vi "test-path-planner-sample.vi"() -> ()   [LabVIEW 2019]
uses:
  <vilib>/Rock Robotics/WPI/ThirdParty/MJansen/PathPlanner/PathPlannerTrajectory.ctl
  <vilib>/Rock Robotics/WPI/ThirdParty/MJansen/PathPlanner/PathPlannerState.ctl
  <vilib>/Rock Robotics/WPI/ThirdParty/JAS_Junk/TrajLib/TypeDef/ROTATION2D.ctl
  <vilib>/Rock Robotics/WPI/ThirdParty/JAS_Junk/TrajLib/TypeDef/TRAJ_STATE.ctl
  <vilib>/Rock Robotics/WPI/ThirdParty/JAS_Junk/TrajLib/TypeDef/POSE2D.ctl
  <vilib>/Rock Robotics/WPI/ThirdParty/JAS_Junk/TrajLib/TypeDef/TRANSLATION2D.ctl
  <vilib>/Rock Robotics/WPI/ThirdParty/MJansen/PathPlanner/PathPlannerWaypoint.ctl
  <vilib>/Rock Robotics/WPI/ThirdParty/JAS_Junk/TrajLib/Util_ApproxEquals.vi
  <vilib>/Rock Robotics/WPI/ThirdParty/MJansen/PathPlanner/PathPlanner.lvlib
  <vilib>/Rock Robotics/WPI/ThirdParty/JAS_Junk/TrajLib/Trajectory_Library.lvlib
  <vilib>/Analysis/NI_AALBase.lvlib
panel:
  in  "Tab Control":T1(tab)
  in  "Max Velocity":dbl=3.0
  in  "Max Acceleration":dbl=2.0
  in  "stop":bool
  in  "Reversed":bool
  out "PathPlannerWayPoints":T2[](array[typedef]) {"HolonomicRotation"."SIN" format="%13.4f"; "HolonomicRotation"."COS" format="%13.4f"; "HolonomicRotation"."VALUE" format="%13.4f"; "NextControl"."Y" format="%14.3f"; "NextControl"."X" format="%14.3f"; "PrevControl"."Y" format="%14.3f"; "PrevControl"."X" format="%14.3f"; "AnchorPoint"."Y" format="%14.3f"; "AnchorPoint"."X" format="%14.3f"}
  in  "Path FileName":string="C:\\Shares\\github\\PathPlannerLabVIEW\\PathPlannerSandbox\\PathPlannerTestPath\\path1.path"
  out "LabVIEW path json read error":errorcluster
  out "PathPlannerTrajectory":T5 {"States"."HolonomicAngular\nvelocity Deg/Sec"."SIN" format="%13.4f"; "States"."HolonomicAngular\nvelocity Deg/Sec"."COS" format="%13.4f"; "States"."HolonomicAngular\nvelocity Deg/Sec"."VALUE" format="%13.4f"; "States"."HolonomicRotation"."SIN" format="%13.4f"; "States"."HolonomicRotation"."COS" format="%13.4f"; "States"."HolonomicRotation"."VALUE" format="%13.4f"; "States"."AngularVelocity"."SIN" format="%13.4f"; "States"."AngularVelocity"."COS" format="%13.4f"; "States"."AngularVelocity"."VALUE" format="%13.4f"; "States"."TrajectoryState"."POSE"."ROTATION"."SIN" format="%13.4f"; "States"."TrajectoryState"."POSE"."ROTATION"."COS" format="%13.4f"; "States"."TrajectoryState"."POSE"."ROTATION"."VALUE" format="%13.4f"; "States"."TrajectoryState"."POSE"."TRANSLATION"."Y" format="%14.3f"; "States"."TrajectoryState"."POSE"."TRANSLATION"."X" format="%14.3f"; "States"."AngularAcceleration"."SIN" format="%13.4f"; "States"."AngularAcceleration"."COS" format="%13.4f"; "States"."AngularAcceleration"."VALUE" format="%13.4f"}
  out "outPathPlannerStates":T6[](array[typedef]) {"HolonomicAngular\nvelocity Deg/Sec"."SIN" format="%13.4f"; "HolonomicAngular\nvelocity Deg/Sec"."COS" format="%13.4f"; "HolonomicAngular\nvelocity Deg/Sec"."VALUE" format="%13.4f"; "HolonomicRotation"."SIN" format="%13.4f"; "HolonomicRotation"."COS" format="%13.4f"; "HolonomicRotation"."VALUE" format="%13.4f"; "AngularVelocity"."SIN" format="%13.4f"; "AngularVelocity"."COS" format="%13.4f"; "AngularVelocity"."VALUE" format="%13.4f"; "TrajectoryState"."POSE"."ROTATION"."SIN" format="%13.4f"; "TrajectoryState"."POSE"."ROTATION"."COS" format="%13.4f"; "TrajectoryState"."POSE"."ROTATION"."VALUE" format="%13.4f"; "TrajectoryState"."POSE"."TRANSLATION"."Y" format="%14.3f"; "TrajectoryState"."POSE"."TRANSLATION"."X" format="%14.3f"; "AngularAcceleration"."SIN" format="%13.4f"; "AngularAcceleration"."COS" format="%13.4f"; "AngularAcceleration"."VALUE" format="%13.4f"}
  in  "index":i32
  out "LabVIEW_TotalTime_Sec":dbl
  out "LabVIEWStateCount":i32
  out "States Check":bool[](array[boolean])
  out "Differences":T7[](array[typedef]) {"POSE"."ROTATION"."SIN" format="%13.4f"; "POSE"."ROTATION"."COS" format="%13.4f"; "POSE"."ROTATION"."VALUE" format="%13.4f"; "POSE"."TRANSLATION"."Y" format="%14.3f"; "POSE"."TRANSLATION"."X" format="%14.3f"}
  out "max time diff":dbl
  out "max vel diff":dbl
  out "max accel diff":dbl
  out "max x diff":dbl
  out "max y diff":dbl
  out "max rot diff rad":dbl
  out "max curvature diff":dbl
  out "vel mean":dbl format="%0.6f"
  out "vel std dev":dbl format="%0.6f"
  out "accel mean":dbl format="%0.6f"
  out "accel std dev":dbl format="%0.6f"
  out "Java and LabVIEW \nwithin tolerance":bool
  out "max accel diff\nindex":i32
  out "max time diff\nindex":i32
  out "Path Samp":T7[](array[typedef]) {"POSE"."ROTATION"."SIN" format="%13.4f"; "POSE"."ROTATION"."COS" format="%13.4f"; "POSE"."ROTATION"."VALUE" format="%13.4f"; "POSE"."TRANSLATION"."Y" format="%14.3f"; "POSE"."TRANSLATION"."X" format="%14.3f"}
  out "LV Samp":T7[](array[typedef]) {"POSE"."ROTATION"."SIN" format="%13.4f"; "POSE"."ROTATION"."COS" format="%13.4f"; "POSE"."ROTATION"."VALUE" format="%13.4f"; "POSE"."TRANSLATION"."Y" format="%14.3f"; "POSE"."TRANSLATION"."X" format="%14.3f"}
  in  "Tolerance":T7={"TimeSeconds"=0.005, "Velocity"=0.005, "Acceleration"=0.2, "POSE"={"TRANSLATION"={"X"=0.002, "Y"=0.002}, "ROTATION"={"VALUE"=0.002, "COS"=0.002, "SIN"=0.002}}, "Curvature"=0.3} {"POSE"."ROTATION"."SIN" format="%13.4f"; "POSE"."ROTATION"."COS" format="%13.4f"; "POSE"."ROTATION"."VALUE" format="%13.4f"; "POSE"."TRANSLATION"."Y" format="%14.3f"; "POSE"."TRANSLATION"."X" format="%14.3f"}
  out "XY SPLINE":cluster{dbl[], dbl[]}[](graph)
  out "XY Graph":cluster{dbl[], dbl[]}[](graph)
  out "Sample Graph":dbl[][](graph)
  out "LabVIEW Time Plot":cluster{dbl[], dbl[]}[](graph)
  out "Diff Time Plot":cluster{dbl[], dbl[]}[](graph)
  in  "PPS2":T6={"AngularAcceleration"={"VALUE"=1.5, "COS"=0.071, "SIN"=0.997}, "PositionMeters"=4.0, "TrajectoryState"={"TimeSeconds"=2.0, "Velocity"=4.0, "Acceleration"=4.0, "POSE"={"TRANSLATION"={"X"=4.0, "Y"=4.0}, "ROTATION"={"VALUE"=1.5, "COS"=0.071, "SIN"=0.997}}, "Curvature"=0.25}, "AngularVelocity"={"VALUE"=1.5, "COS"=0.071, "SIN"=0.997}, "HolonomicRotation"={"VALUE"=1.5, "COS"=0.071, "SIN"=0.997}, "CurveRadius"=4.0, "DeltaPos"=2.0, "HolonomicAngular\nvelocity Deg/Sec"={"VALUE"=0.0, "COS"=1.0, "SIN"=0.0}} {"HolonomicAngular\nvelocity Deg/Sec"."SIN" format="%13.4f"; "HolonomicAngular\nvelocity Deg/Sec"."COS" format="%13.4f"; "HolonomicAngular\nvelocity Deg/Sec"."VALUE" format="%13.4f"; "HolonomicRotation"."SIN" format="%13.4f"; "HolonomicRotation"."COS" format="%13.4f"; "HolonomicRotation"."VALUE" format="%13.4f"; "AngularVelocity"."SIN" format="%13.4f"; "AngularVelocity"."COS" format="%13.4f"; "AngularVelocity"."VALUE" format="%13.4f"; "TrajectoryState"."POSE"."ROTATION"."SIN" format="%13.4f"; "TrajectoryState"."POSE"."ROTATION"."COS" format="%13.4f"; "TrajectoryState"."POSE"."ROTATION"."VALUE" format="%13.4f"; "TrajectoryState"."POSE"."TRANSLATION"."Y" format="%14.3f"; "TrajectoryState"."POSE"."TRANSLATION"."X" format="%14.3f"; "AngularAcceleration"."SIN" format="%13.4f"; "AngularAcceleration"."COS" format="%13.4f"; "AngularAcceleration"."VALUE" format="%13.4f"}
  in  "PPS1":T6={"AngularAcceleration"={"VALUE"=0.5, "COS"=0.878, "SIN"=0.479}, "PositionMeters"=2.0, "TrajectoryState"={"TimeSeconds"=1.0, "Velocity"=2.0, "Acceleration"=2.0, "POSE"={"TRANSLATION"={"X"=2.0, "Y"=2.0}, "ROTATION"={"VALUE"=0.5, "COS"=0.878, "SIN"=0.479}}, "Curvature"=0.5}, "AngularVelocity"={"VALUE"=0.0, "COS"=1.0, "SIN"=0.0}, "HolonomicRotation"={"VALUE"=0.5, "COS"=0.878, "SIN"=0.479}, "CurveRadius"=2.0, "DeltaPos"=1.0, "HolonomicAngular\nvelocity Deg/Sec"={"VALUE"=0.0, "COS"=1.0, "SIN"=0.0}} {"HolonomicAngular\nvelocity Deg/Sec"."SIN" format="%13.4f"; "HolonomicAngular\nvelocity Deg/Sec"."COS" format="%13.4f"; "HolonomicAngular\nvelocity Deg/Sec"."VALUE" format="%13.4f"; "HolonomicRotation"."SIN" format="%13.4f"; "HolonomicRotation"."COS" format="%13.4f"; "HolonomicRotation"."VALUE" format="%13.4f"; "AngularVelocity"."SIN" format="%13.4f"; "AngularVelocity"."COS" format="%13.4f"; "AngularVelocity"."VALUE" format="%13.4f"; "TrajectoryState"."POSE"."ROTATION"."SIN" format="%13.4f"; "TrajectoryState"."POSE"."ROTATION"."COS" format="%13.4f"; "TrajectoryState"."POSE"."ROTATION"."VALUE" format="%13.4f"; "TrajectoryState"."POSE"."TRANSLATION"."Y" format="%14.3f"; "TrajectoryState"."POSE"."TRANSLATION"."X" format="%14.3f"; "AngularAcceleration"."SIN" format="%13.4f"; "AngularAcceleration"."COS" format="%13.4f"; "AngularAcceleration"."VALUE" format="%13.4f"}
  in  "PPS0":T6={"AngularAcceleration"={"VALUE"=0.0, "COS"=1.0, "SIN"=0.0}, "PositionMeters"=1.0, "TrajectoryState"={"TimeSeconds"=0.0, "Velocity"=1.0, "Acceleration"=1.0, "POSE"={"TRANSLATION"={"X"=1.0, "Y"=1.0}, "ROTATION"={"VALUE"=0.0, "COS"=1.0, "SIN"=0.0}}, "Curvature"=1.0}, "AngularVelocity"={"VALUE"=0.0, "COS"=1.0, "SIN"=0.0}, "HolonomicRotation"={"VALUE"=0.0, "COS"=1.0, "SIN"=0.0}, "CurveRadius"=1.0, "DeltaPos"=1.0, "HolonomicAngular\nvelocity Deg/Sec"={"VALUE"=0.0, "COS"=1.0, "SIN"=0.0}} {"HolonomicAngular\nvelocity Deg/Sec"."SIN" format="%13.4f"; "HolonomicAngular\nvelocity Deg/Sec"."COS" format="%13.4f"; "HolonomicAngular\nvelocity Deg/Sec"."VALUE" format="%13.4f"; "HolonomicRotation"."SIN" format="%13.4f"; "HolonomicRotation"."COS" format="%13.4f"; "HolonomicRotation"."VALUE" format="%13.4f"; "AngularVelocity"."SIN" format="%13.4f"; "AngularVelocity"."COS" format="%13.4f"; "AngularVelocity"."VALUE" format="%13.4f"; "TrajectoryState"."POSE"."ROTATION"."SIN" format="%13.4f"; "TrajectoryState"."POSE"."ROTATION"."COS" format="%13.4f"; "TrajectoryState"."POSE"."ROTATION"."VALUE" format="%13.4f"; "TrajectoryState"."POSE"."TRANSLATION"."Y" format="%14.3f"; "TrajectoryState"."POSE"."TRANSLATION"."X" format="%14.3f"; "AngularAcceleration"."SIN" format="%13.4f"; "AngularAcceleration"."COS" format="%13.4f"; "AngularAcceleration"."VALUE" format="%13.4f"}
  out "TrajState":T7={"TimeSeconds"=0.0, "Velocity"=0.0, "Acceleration"=0.0, "POSE"={"TRANSLATION"={"X"=0.0, "Y"=0.0}, "ROTATION"={"VALUE"=0.0, "COS"=1.0, "SIN"=0.0}}, "Curvature"=0.0} {"POSE"."ROTATION"."SIN" format="%13.4f"; "POSE"."ROTATION"."COS" format="%13.4f"; "POSE"."ROTATION"."VALUE" format="%13.4f"; "POSE"."TRANSLATION"."Y" format="%14.3f"; "POSE"."TRANSLATION"."X" format="%14.3f"}
  out "PathState":T7={"TimeSeconds"=0.0, "Velocity"=0.0, "Acceleration"=0.0, "POSE"={"TRANSLATION"={"X"=0.0, "Y"=0.0}, "ROTATION"={"VALUE"=0.0, "COS"=1.0, "SIN"=0.0}}, "Curvature"=0.0} {"POSE"."ROTATION"."SIN" format="%13.4f"; "POSE"."ROTATION"."COS" format="%13.4f"; "POSE"."ROTATION"."VALUE" format="%13.4f"; "POSE"."TRANSLATION"."Y" format="%14.3f"; "POSE"."TRANSLATION"."X" format="%14.3f"}
  out "LabVIEWStates":T7[](array[typedef]) {"POSE"."ROTATION"."SIN" format="%13.4f"; "POSE"."ROTATION"."COS" format="%13.4f"; "POSE"."ROTATION"."VALUE" format="%13.4f"; "POSE"."TRANSLATION"."Y" format="%14.3f"; "POSE"."TRANSLATION"."X" format="%14.3f"}
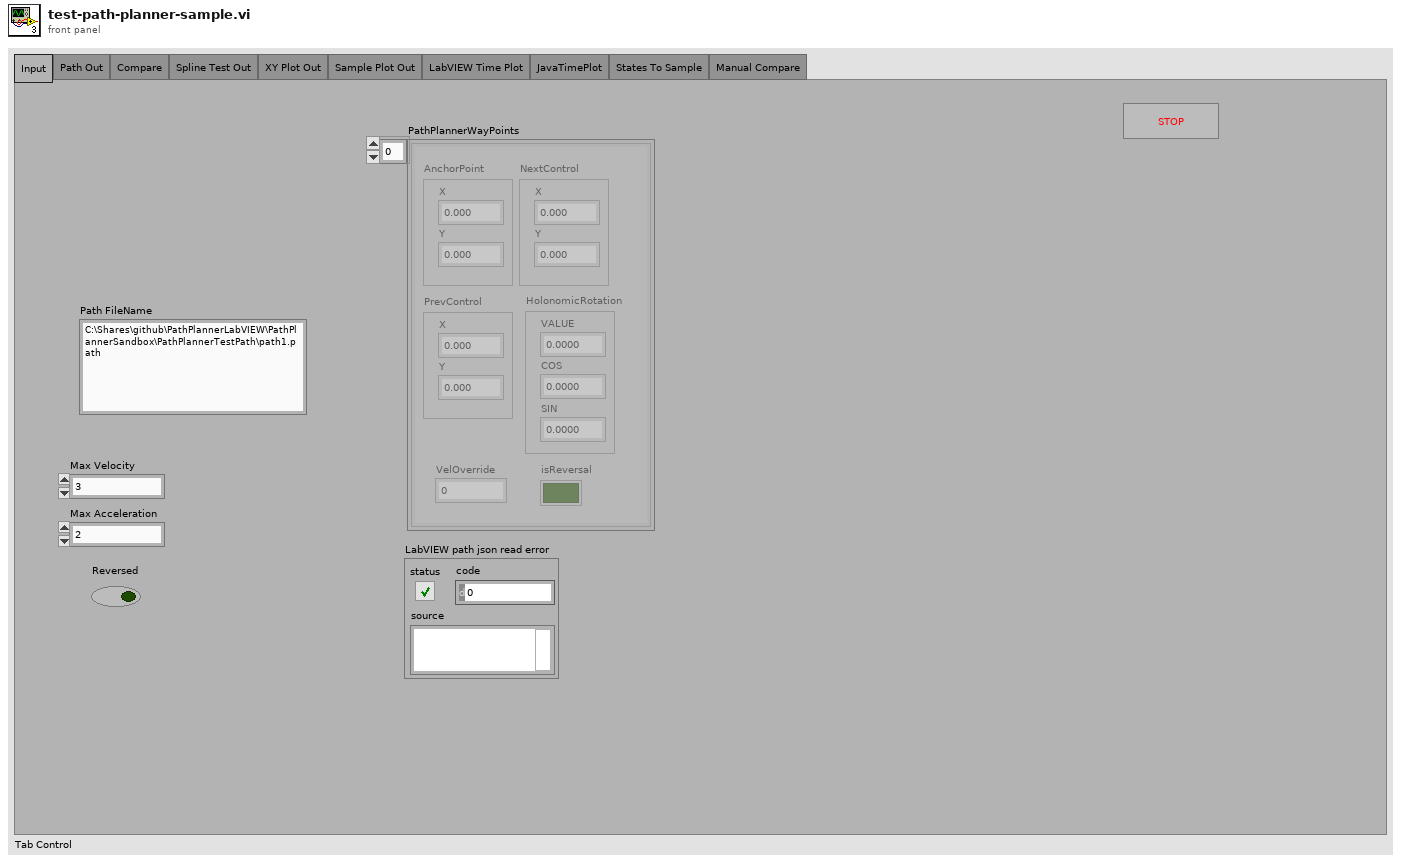
[diagram p1: front panel]
types:
  T1 = enum32{"Input", "Path Out", "Compare", "Spline Test Out", "XY Plot Out", "Sample Plot Out", "LabVIEW Time Plot", "JavaTimePlot", "States To Sample", "Manual Compare"}
  T2 = typedef "PathPlanner.lvlib/PathPlannerWaypoint.ctl" = cluster{"AnchorPoint":T3, "PrevControl":T3, "NextControl":T3, "HolonomicRotation":T4, "VelOverride":dbl, "isReversal":bool}
  T3 = typedef "Trajectory_Library.lvlib/TRANSLATION2D.ctl" = cluster{"X":dbl, "Y":dbl}
  T4 = typedef "Trajectory_Library.lvlib/ROTATION2D.ctl" = cluster{"VALUE":dbl, "COS":dbl, "SIN":dbl}
  T5 = typedef "PathPlanner.lvlib/PathPlannerTrajectory.ctl" = cluster{"TotalTimeSeconds":dbl, "States":T6[]}
  T6 = typedef "PathPlanner.lvlib/PathPlannerState.ctl" = cluster{"AngularAcceleration":T4, "PositionMeters":dbl, "TrajectoryState":T7, "AngularVelocity":T4, "HolonomicRotation":T4, "CurveRadius":dbl, "DeltaPos":dbl, "HolonomicAngular\nvelocity Deg/Sec":T4}
  T7 = typedef "Trajectory_Library.lvlib/TRAJ_STATE.ctl" = cluster{"TimeSeconds":dbl, "Velocity":dbl, "Acceleration":dbl, "POSE":T8, "Curvature":dbl}
  T8 = typedef "Trajectory_Library.lvlib/POSE2D.ctl" = cluster{"TRANSLATION":T3, "ROTATION":T4}
  T9 = typedef "Trajectory_Library.lvlib/TRAJECTORY.ctl" = cluster{"TotalTImeSecs":dbl, "States":T7[]}
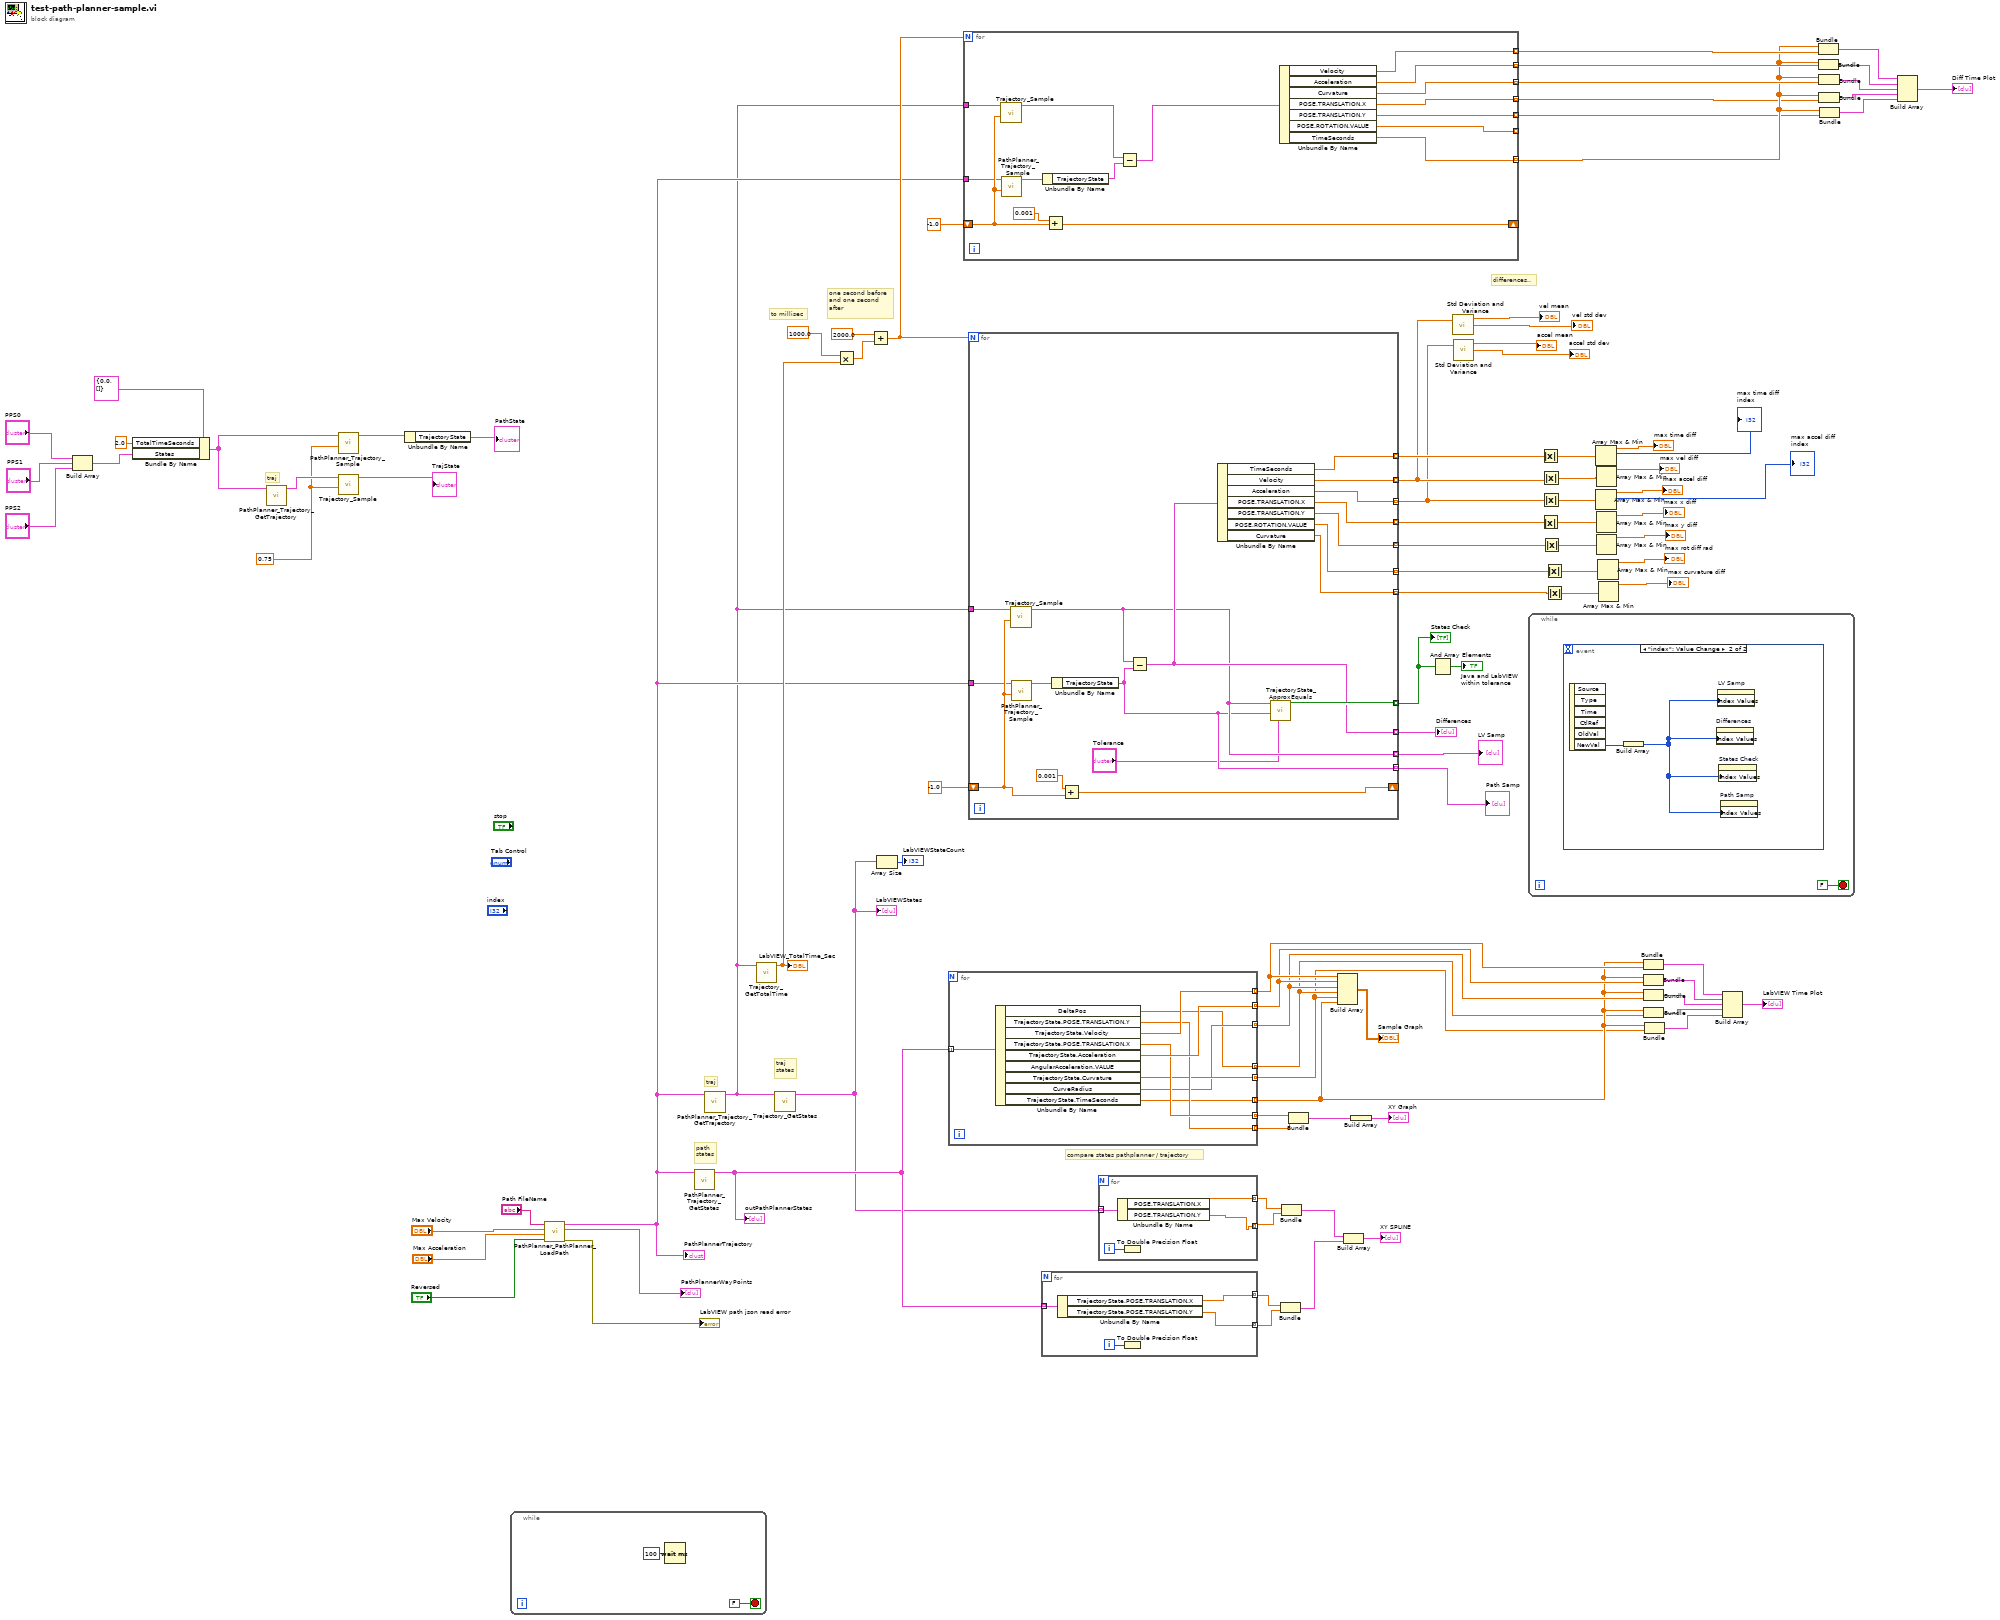
[diagram p0: block diagram]
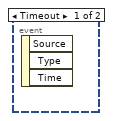
[diagram p2: hidden frame]
diagram:
  w8 = 0.75
  # "traj"
  # "one second before\nand one second\nafter"
  # "to millisec"
  # "compare states pathplanner / trajectory"
  # "traj"
  # "traj\nstates"
  # "path\nstates"
  # "differences.."
  n1 = Build Array("PPS0", "PPS1", "PPS2") -> (w12:T6[])
  n2 = Bundle By Name(cluster=T5 {"TotalTimeSeconds"=0.0, "States"=[]} ("PathPlannerTrajectory"), "TotalTimeSeconds"=2.0, "States"=w12) -> (w10:T5)
  n3 = call <vilib>:"PathPlanner_Trajectory_GetTrajectory.vi"("PathPlannerTrajectory"=w10) -> ("TRAJECTORY"=w9:T9)  [unwired: 10 in]
  n4 = call <vilib>:"PathPlanner_Trajectory_Sample.vi"("Time"=w8, "PathPlannerTrajectory"=w10) -> ("PathPlannerState"=w6:T6)  [unwired: 9 in]
  n5 = call <vilib>:"Trajectory_Sample.vi"("Time"=w8, "InputTRAJECTORY"=w9) -> ("OutputTRAJ_STATE"=→"TrajState":T7)  [unwired: 9 in]
  n6 = Unbundle By Name(w6) -> ("TrajectoryState"=→"PathState":T7)
  n7 = while {
    stop <- FALSE stop-if-true
    n8 = Wait (ms)(milliseconds to wait=u32 100) -> ()  [unwired: 1 out]
  }
  n9 = call <vilib>:"PathPlanner_PathPlanner_LoadPath.vi"("Reversed"="Reversed", "MaxAcceleration"="Max Acceleration", "MaxVelocity"="Max Velocity", "FileName"="Path FileName") -> ("error out"=→"LabVIEW path json read error":errorcluster, "PathPlannerWayPoints"=→"PathPlannerWayPoints":T2[], "PathPlannerTrajectory"=w33:T5)  [unwired: 4 in, 1 out]
  "PathPlannerTrajectory" <- w33
  n10 = call <vilib>:"PathPlanner_Trajectory_GetStates.vi"("PathPlannerTrajectory"=w33) -> ("PathPlannerStates"=w79:T6[])  [unwired: 10 in]
  "outPathPlannerStates" <- w79
  n11 = call <vilib>:"PathPlanner_Trajectory_GetTrajectory.vi"("PathPlannerTrajectory"=w33) -> ("TRAJECTORY"=w32:T9)  [unwired: 10 in]
  n12 = call <vilib>:"Trajectory_GetTotalTime.vi"("TRAJECTORY"=w32) -> ("TotalTime_Sec"=w36:dbl)  [unwired: 10 in]
  "LabVIEW_TotalTime_Sec" <- w36
  n13 = call <vilib>:"Trajectory_GetStates.vi"("TRAJECTORY"=w32) -> ("States"=w37:T7[])  [unwired: 10 in]
  "LabVIEWStates" <- w37
  n14 = Multiply(x=1000.0, y=w36) -> (x*y=w40:dbl)
  n15 = Add(x=2000.0, y=w40) -> (x+y=w35:dbl)
  n16 = Array Size(array=w37) -> (size(s)=→"LabVIEWStateCount":i32)
  n17 = for {
    tunnel: [w109] -> w66 mode=indexing
    tunnel: [w108] -> w65 mode=indexing
    tunnel: [w102] -> w62 mode=indexing
    tunnel: [w107] -> w97 mode=indexing
    tunnel: [w106] -> w96 mode=indexing
    tunnel: w79 -> [w105] mode=indexing
    tunnel: [w104] -> w61 mode=indexing
    tunnel: [w103] -> w64 mode=indexing
    tunnel: [w101] -> w63 mode=indexing
    n18 = Unbundle By Name(w105) -> ("DeltaPos"=w102:dbl, "TrajectoryState.POSE.TRANSLATION.Y"=w106:dbl, "TrajectoryState.Velocity"=w109:dbl, "TrajectoryState.POSE.TRANSLATION.X"=w107:dbl, "TrajectoryState.Acceleration"=w108:dbl, "TrajectoryState.Curvature"=w104:dbl, "CurveRadius"=w103:dbl, "TrajectoryState.TimeSeconds"=w101:dbl)  [unwired: 1 out]
  }
  n19 = for {
    N: w35 -> [_]
    tunnel: [w115] -> w55 mode=indexing
    tunnel: [w114] -> w54 mode=indexing
    tunnel: [w112] -> w51 mode=indexing
    tunnel: [w111] -> w50 mode=indexing
    tunnel: [w113] -> w53 mode=indexing
    tunnel: [w125] -> w52 mode=indexing
    shift-right: [w119] -> _
    shift-left: -1.0 -> [w118]
    tunnel: w33 -> [w117]
    tunnel: w32 -> [w116]
    tunnel: [w110] -> _ mode=indexing
    n20 = call <vilib>:"Trajectory_Sample.vi"("Time"=w118, "InputTRAJECTORY"=w116) -> ("OutputTRAJ_STATE"=w123:T7)  [unwired: 9 in]
    n21 = call <vilib>:"PathPlanner_Trajectory_Sample.vi"("Time"=w118, "PathPlannerTrajectory"=w117) -> ("PathPlannerState"=w124:T6)  [unwired: 9 in]
    n22 = Unbundle By Name(w124) -> ("TrajectoryState"=w122:T7)
    n23 = Add(x=0.001, y=w118) -> (x+y=w119:dbl)
    n24 = Subtract(x=w123, y=w122) -> (x-y=w121:T7)
    n25 = Unbundle By Name(w121) -> ("Velocity"=w115:dbl, "Acceleration"=w114:dbl, "Curvature"=w113:dbl, "POSE.TRANSLATION.X"=w112:dbl, "POSE.TRANSLATION.Y"=w111:dbl, "POSE.ROTATION.VALUE"=w110:dbl, "TimeSeconds"=w125:dbl)
  }
  n26 = for {
    N: w35 -> [_]
    tunnel: [w143] -> w44 mode=indexing
    tunnel: [w142] -> w31 mode=indexing
    tunnel: [w141] -> w18 mode=indexing
    tunnel: [w140] -> w17 mode=indexing
    tunnel: [w139] -> w30 mode=indexing
    tunnel: [w138] -> w29 mode=indexing
    tunnel: [w137] -> w28 mode=indexing
    tunnel: [w136] -> w27 mode=indexing
    shift-right: [w134] -> _
    shift-left: -1.0 -> [w132]
    tunnel: w33 -> [w131]
    tunnel: w32 -> [w130]
    tunnel: [w129] -> w19 mode=indexing
    tunnel: [w128] -> w2 mode=indexing
    tunnel: [w127] -> w1 mode=indexing
    n27 = call <vilib>:"Trajectory_Sample.vi"("Time"=w132, "InputTRAJECTORY"=w130) -> ("OutputTRAJ_STATE"=w128:T7)  [unwired: 9 in]
    n28 = call <vilib>:"PathPlanner_Trajectory_Sample.vi"("Time"=w132, "PathPlannerTrajectory"=w131) -> ("PathPlannerState"=w133:T6)  [unwired: 9 in]
    n29 = Unbundle By Name(w133) -> ("TrajectoryState"=w127:T7)
    n30 = Add(x=0.001, y=w132) -> (x+y=w134:dbl)
    n31 = Subtract(x=w128, y=w127) -> (x-y=w129:T7)
    n32 = Unbundle By Name(w129) -> ("TimeSeconds"=w142:dbl, "Velocity"=w141:dbl, "Acceleration"=w140:dbl, "POSE.TRANSLATION.X"=w139:dbl, "POSE.TRANSLATION.Y"=w138:dbl, "POSE.ROTATION.VALUE"=w137:dbl, "Curvature"=w136:dbl)
    n33 = call "TrajectoryState_ApproxEquals.vi"("Tolerance"="Tolerance", "Other TRAJ_STATE"=w127, "TRAJ_STATE"=w128) -> ("Equals"=w143:bool)  [unwired: 8 in]
  }
  "States Check" <- w44
  "Differences" <- w19
  "LV Samp" <- w2
  "Path Samp" <- w1
  n34 = for {
    tunnel: [w146] -> w91 mode=indexing
    tunnel: w79 -> [w145] mode=indexing
    tunnel: [w144] -> w90 mode=indexing
    i -> [w147]
    n35 = Unbundle By Name(w145) -> ("TrajectoryState.POSE.TRANSLATION.X"=w146:dbl, "TrajectoryState.POSE.TRANSLATION.Y"=w144:dbl)
    n36 = To Double Precision Float(number=w147) -> ()  [unwired: 1 out]
  }
  n37 = for {
    tunnel: [w150] -> w93 mode=indexing
    tunnel: [w149] -> w92 mode=indexing
    tunnel: w37 -> [w148] mode=indexing
    i -> [w151]
    n38 = Unbundle By Name(w148) -> ("POSE.TRANSLATION.X"=w150:dbl, "POSE.TRANSLATION.Y"=w149:dbl)
    n39 = To Double Precision Float(number=w151) -> ()  [unwired: 1 out]
  }
  n40 = Bundle(w91, w90) -> (w88:cluster{dbl[], dbl[]})  [unwired: 1 in]
  n41 = Bundle(w93, w92) -> (w89:cluster{dbl[], dbl[]})  [unwired: 1 in]
  n42 = Bundle(w97, w96) -> (w95:cluster{dbl[], dbl[]})  [unwired: 1 in]
  n43 = Build Array(w66, w65, w64, w62, w61, w63) -> (→"Sample Graph":dbl[][])
  n44 = Build Array(w89, w88) -> (→"XY SPLINE":cluster{dbl[], dbl[]}[])
  n45 = Build Array(w95) -> (→"XY Graph":cluster{dbl[], dbl[]}[])
  n46 = And Array Elements(Boolean array=w44) -> (logical AND=→"Java and LabVIEW \nwithin tolerance":bool)
  n47 = call <vilib>:"Std Deviation and Variance.vi"("X"=w18) -> ("mean"=→"vel mean":dbl, "standard deviation"=→"vel std dev":dbl)  [unwired: 1 in, 1 out]
  n48 = call <vilib>:"Std Deviation and Variance.vi"("X"=w17) -> ("mean"=→"accel mean":dbl, "standard deviation"=→"accel std dev":dbl)  [unwired: 1 in, 1 out]
  n49 = while {
    stop <- FALSE stop-if-true
    n50 = event shown="[1] \"index\": Value Change" {
      selector: _ -> [_ _]
      dyn-events: _ -> [_ _]
      timeout: _ -> [_ _]
      event Timeout {
        n51 = event-data() -> ()  [unwired: 1 in, 3 out]
      }
      event "index": Value Change {
        n52 = event-data() -> ("NewVal"=w154:i32)  [unwired: 1 in, 5 out]
        n53 = Build Array(w154) -> (w153:i32[])
        n54 = property on="Differences" class="Arr (strict)"("Index Values"=w153) -> ()  [unwired: 2 in, 2 out]
        n55 = property on="LV Samp" class="Arr (strict)"("Index Values"=w153) -> ()  [unwired: 2 in, 2 out]
        n56 = property on="States Check" class="Arr (strict)"("Index Values"=w153) -> ()  [unwired: 2 in, 2 out]
        n57 = property on="Path Samp" class="Arr (strict)"("Index Values"=w153) -> ()  [unwired: 2 in, 2 out]
      }
    }
  }
  n58 = Absolute Value(x=w31) -> (abs(x)=w26:dbl[])
  n59 = Absolute Value(x=w30) -> (abs(x)=w23:dbl[])
  n60 = Absolute Value(x=w18) -> (abs(x)=w25:dbl[])
  n61 = Absolute Value(x=w17) -> (abs(x)=w24:dbl[])
  n62 = Absolute Value(x=w29) -> (abs(x)=w22:dbl[])
  n63 = Absolute Value(x=w28) -> (abs(x)=w21:dbl[])
  n64 = Absolute Value(x=w27) -> (abs(x)=w20:dbl[])
  n65 = Array Max & Min(array=w26) -> (max value=→"max time diff":dbl, max index (indices)=→"max time diff\nindex":i32)  [unwired: 2 out]
  n66 = Array Max & Min(array=w24) -> (max value=→"max accel diff":dbl, max index (indices)=→"max accel diff\nindex":i32)  [unwired: 2 out]
  n67 = Array Max & Min(array=w25) -> (max value=→"max vel diff":dbl)  [unwired: 3 out]
  n68 = Array Max & Min(array=w23) -> (max value=→"max x diff":dbl)  [unwired: 3 out]
  n69 = Array Max & Min(array=w22) -> (max value=→"max y diff":dbl)  [unwired: 3 out]
  n70 = Array Max & Min(array=w21) -> (max value=→"max rot diff rad":dbl)  [unwired: 3 out]
  n71 = Array Max & Min(array=w20) -> (max value=→"max curvature diff":dbl)  [unwired: 3 out]
  n72 = Bundle(w63, w66) -> (w60:cluster{dbl[], dbl[]})  [unwired: 1 in]
  n73 = Bundle(w63, w65) -> (w59:cluster{dbl[], dbl[]})  [unwired: 1 in]
  n74 = Bundle(w63, w64) -> (w58:cluster{dbl[], dbl[]})  [unwired: 1 in]
  n75 = Bundle(w63, w62) -> (w57:cluster{dbl[], dbl[]})  [unwired: 1 in]
  n76 = Bundle(w63, w61) -> (w56:cluster{dbl[], dbl[]})  [unwired: 1 in]
  n77 = Build Array(w60, w59, w58, w57, w56) -> (→"LabVIEW Time Plot":cluster{dbl[], dbl[]}[])
  n78 = Bundle(w52, w55) -> (w49:cluster{dbl[], dbl[]})  [unwired: 1 in]
  n79 = Bundle(w52, w54) -> (w48:cluster{dbl[], dbl[]})  [unwired: 1 in]
  n80 = Bundle(w52, w53) -> (w47:cluster{dbl[], dbl[]})  [unwired: 1 in]
  n81 = Bundle(w52, w51) -> (w46:cluster{dbl[], dbl[]})  [unwired: 1 in]
  n82 = Bundle(w52, w50) -> (w45:cluster{dbl[], dbl[]})  [unwired: 1 in]
  n83 = Build Array(w49, w48, w47, w46, w45) -> (→"Diff Time Plot":cluster{dbl[], dbl[]}[])
